vi "Do.vi"(8 "error in (no error)":errorcluster, 10 "Context in":refnum<data-value>, 11 "Active in":refnum<class "Active.lvclass">) -> (0 "error out":errorcluster, 2 "Context out":refnum<data-value>, 3 "Active out":refnum<class "Active.lvclass">)   [LabVIEW 2024]
uses:
  Active.lvclass/Active.ctl
  Context/Context/Context.lvclass
  Active.lvclass
panel:
  out "Numeric":dbl
  # "DO!"
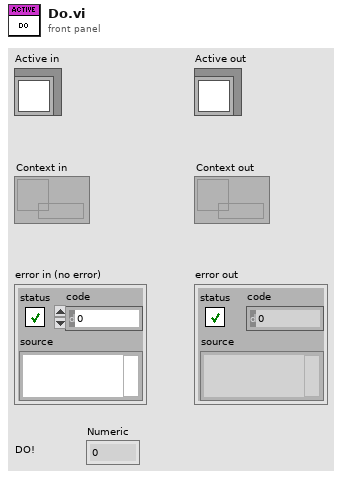
[diagram p1: front panel]
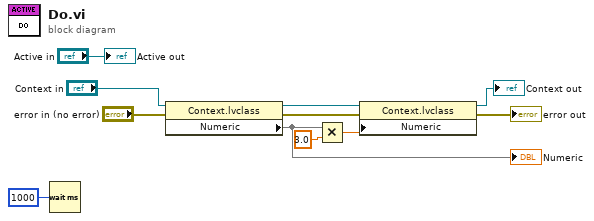
[diagram p0: block diagram]
diagram:
  n1 = Wait (ms)(milliseconds to wait=u32 1000) -> ()  [unwired: 1 out]
  n2 = property class="Context.lvclass"(reference="Context in", error in="error in (no error)") -> (reference out=w7:refnum<data-value>, error out=w4:errorcluster, "Numeric"=w1)
  "Numeric" <- w1
  n3 = Multiply(x=w1, y=3.0) -> (x*y=w6:dbl)
  n4 = property class="Context.lvclass"(reference=w7, error in=w4, "Numeric"=w6) -> (reference out=→"Context out":refnum<data-value>, error out=→"error out":errorcluster)
  "Active out" <- "Active in"
